vi "Write normFactor.vi"(8 "error in (no error)":errorcluster, 10 "normFactor":dbl, 11 "AlignSkill in":refnum<class "AlignSkill.lvclass">) -> (0 "error out":errorcluster, 3 "AlignSkill out":refnum<class "AlignSkill.lvclass">)   [LabVIEW 2023, in "AlignSkill.lvclass"]
uses:
  AlignSkill.lvclass
  AlignSkill.lvclass/AlignSkill.ctl
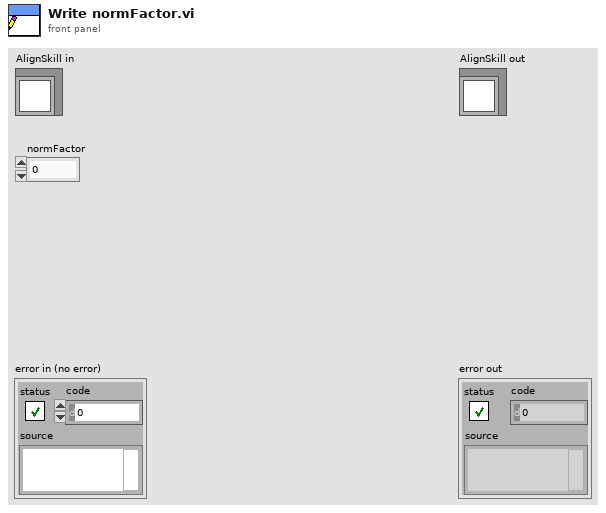
[diagram p1: front panel]
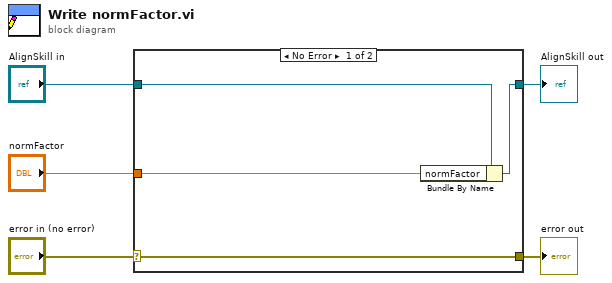
[diagram p0: block diagram]
diagram:
  n1 = case shown="No Error" "error in (no error)" {
    selector: "error in (no error)" -> [w9 w10]
    tunnel: [w9 w10] -> w4
    tunnel: [w7 w11] -> w2
    tunnel: "AlignSkill in" -> [w8 w11]
    tunnel: "normFactor" -> [w6 _]
    frame No Error {
      n2 = Bundle By Name(cluster=w8, "normFactor"=w6) -> (w7:refnum<class "AlignSkill.lvclass">)
    }
    frame Error {
    }
  }
  "error out" <- w4
  "AlignSkill out" <- w2
